vi "Begin.vi"(8 "error in":errorcluster) -> (0 "error out":errorcluster)   [LabVIEW 2019]
doc: "Called before other user functions, this VI is expected to open initial I/O refnums, load in file data, and do all program initialization. Notice that the <B>error out</B> terminal is simply used for data flow. Wiring it to other structures or subVIs ensures that this VI runs first."
uses:
  <vilib>/Rock Robotics/WPI/DriverStation/WPI_DriverStationRobotMode2.ctl
  <vilib>/Rock Robotics/WPI/Joystick/WPI_JoystickDeviceEnum.ctl
  Robot Global Data.vi
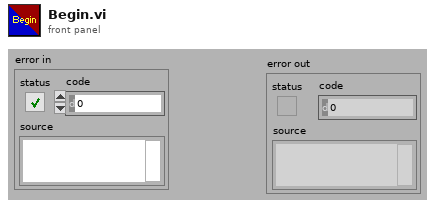
[diagram p1: front panel]
types:
  T1 = typedef "WPI_JoystickDeviceEnum.ctl" = enum16{"USB 0", "USB 1", "USB 2", "USB 3", "USB 4", "USB 5"}
  T2 = typedef "WPI_DriverStationRobotMode2.ctl" = enum16{"Autonomous Disabled", "Autonomous Enabled", "Teleop Disabled", "Teleop Enabled", "Disconnected", "Finish", "Test Disabled", "Test Enabled", "Emergency Stopped"}
  T3 = typedef "WPI_JoystickDevRef.ctl" = cluster{"Device":T1}
  T4 = typedef "WPI_MotorControlDeviceRef.ctl" = cluster{"DeviceStatus":errorcluster, "Type":T5, "PWM":cluster{"PWM Channel":T6, "DeadBand":T7}, "CAN":cluster{"Device Number":u8, "SetOutput VI Ref":variant, "GetOutput VI Ref":variant, "Enable VI Ref":variant, "Disable VI Ref":variant, "Data":variant}, "Invert":bool, "DIO PWM":cluster{"PWM \"Enable\" Channel":T6, "DIOChannel":T8, "PWM Rate":dbl}}
  T5 = typedef "WPI_MotorControlType.ctl" = enum16{"PWM", "CAN", "DIO PWM"}
  T6 = typedef "FPGA_DIOPWMChannel.ctl" = enum8{"PWM 0", "PWM 1", "PWM 2", "PWM 3", "PWM 4", "PWM 5", "PWM 6", "PWM 7", "PWM 8", "PWM 9", "PWM MXP 0", "PWM MXP 1", "PWM MXP 2", "PWM MXP 3", "PWM MXP 4", "PWM MXP 5", "PWM MXP 6", "PWM MXP 7", "PWM MXP 8", "PWM MXP 9", "Invalid"}
  T7 = typedef "WPI_PWMDeadband.ctl" = cluster{"Name":string, "maxPositivePwm":i32, "minPositivePwm":i32, "centerPwm":i32, "maxNegativePwm":i32, "minNegativePwm":i32, "angularRange":u16}
  T8 = typedef "FPGA_DIOChannel.ctl" = enum8{"DIO 0", "DIO 1", "DIO 2", "DIO 3", "DIO 4", "DIO 5", "DIO 6", "DIO 7", "DIO 8", "DIO 9", "DIO MXP 0", "DIO MXP 1", "DIO MXP 2", "DIO MXP 3", "DIO MXP 4", "DIO MXP 5", "DIO MXP 6", "DIO MXP 7", "DIO MXP 8", "DIO MXP 9", "DIO MXP 10", "DIO MXP 11", "DIO MXP 12", "DIO MXP 13", "DIO MXP 14", "DIO MXP 15", "SPI Port CS1", "SPI Port CS2", "SPI Port CS3", "SPI Port MISO", "SPI Port MOSI", "Invalid"}
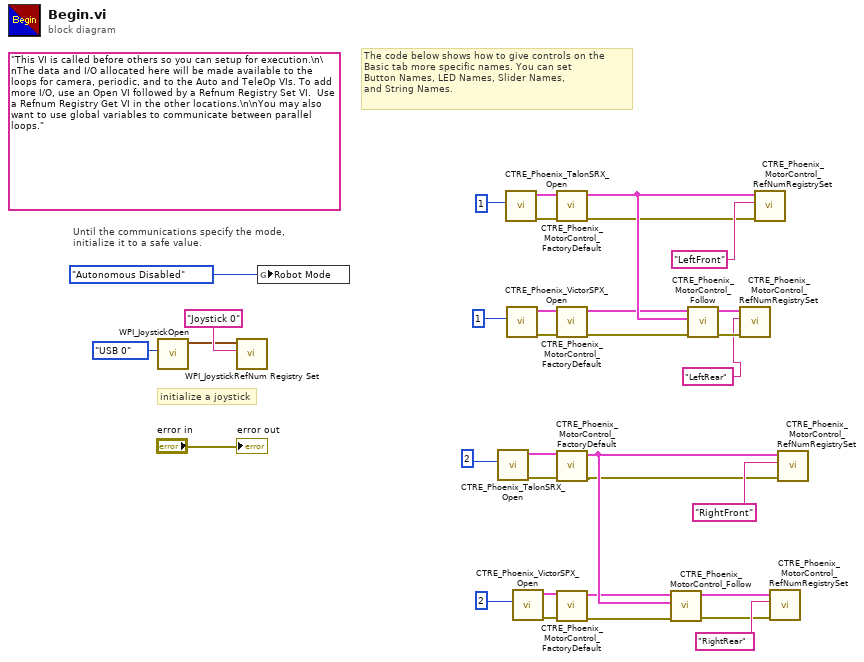
[diagram p0: block diagram]
diagram:
  (unwired) "This VI is called before others so you can setup for execution.\n\nThe data and I/O allocated here will be made available to the loops for camera, periodic, and to the Auto and TeleOp VIs. To add more I/O, use an Open VI followed by a Refnum Registry Set VI.  Use a Refnum Registry Get VI in the other locations.\n\nYou may also want to use global variables to communicate between parallel loops."
  # "The code below shows how to give controls on the\nBasic tab more specific names. You can set\nButton Names, LED Names, Slider Names,\nand String Names."
  # "initialize a joystick"
  # "Until the communications specify the mode,\ninitialize it to a safe value."
  n1 = call <vilib>:"WPI_JoystickOpen.vi"("JoystickDevice"=WPI_JoystickDeviceEnum."USB 0") -> ("JoystickDevRef"=w32:T3)  [unwired: 10 in]
  n2 = call <vilib>:"WPI_JoystickRefNum Registry Set.vi"("refnum name"="Joystick 0", "JoystickDevRef"=w32) -> ()  [unwired: 8 in, 2 out]
  n3 = global write "Robot Global Data.vi" "Robot Mode"(WPI_DriverStationRobotMode2."Autonomous Disabled" ("Robot Mode")) -> ()
  n4 = call <vilib>:"CTRE_Phoenix_TalonSRX_Open.vi"("Device Number"=u8 2) -> ("error out"=w5:errorcluster, "CAN Talon SRX Ref"=w15:T4)  [unwired: 9 in]
  n5 = call <vilib>:"CTRE_Phoenix_TalonSRX_Open.vi"("Device Number"=u8 1) -> ("error out"=w7:errorcluster, "CAN Talon SRX Ref"=w17:T4)  [unwired: 9 in]
  n6 = call <vilib>:"CTRE_Phoenix_VictorSPX_Open.vi"("Device Number"=u8 1) -> ("error out"=w9:errorcluster, "CAN Talon SRX Ref"=w11:T4)  [unwired: 9 in]
  n7 = call <vilib>:"CTRE_Phoenix_VictorSPX_Open.vi"("Device Number"=u8 2) -> ("error out"=w3:errorcluster, "CAN Talon SRX Ref"=w13:T4)  [unwired: 9 in]
  n8 = call <vilib>:"CTRE_Phoenix_MotorControl_FactoryDefault.vi"("error in"=w7, "PhoenixMotorControlDevRef"=w17) -> ("error out"=w6:errorcluster, "PhoenixMotorControlDevRef"=w16:T4)  [unwired: 8 in]
  n9 = call <vilib>:"CTRE_Phoenix_MotorControl_FactoryDefault.vi"("error in"=w9, "PhoenixMotorControlDevRef"=w11) -> ("error out"=w8:errorcluster, "PhoenixMotorControlDevRef"=w10:T4)  [unwired: 8 in]
  n10 = call <vilib>:"CTRE_Phoenix_MotorControl_FactoryDefault.vi"("error in"=w5, "PhoenixMotorControlDevRef"=w15) -> ("error out"=w4:errorcluster, "PhoenixMotorControlDevRef"=w14:T4)  [unwired: 8 in]
  n11 = call <vilib>:"CTRE_Phoenix_MotorControl_FactoryDefault.vi"("error in"=w3, "PhoenixMotorControlDevRef"=w13) -> ("error out"=w2:errorcluster, "PhoenixMotorControlDevRef"=w12:T4)  [unwired: 8 in]
  n12 = call <vilib>:"CTRE_Phoenix_MotorControl_Follow.vi"("error in (no error)"=w2, "Master Controller to Follow"=w14, "PhoenixMotorControlDevRef"=w12) -> ("error out"=w19:errorcluster, "PhoenixMotorControlDevRef"=w18:T4)  [unwired: 7 in]
  n13 = call <vilib>:"CTRE_Phoenix_MotorControl_Follow.vi"("error in (no error)"=w8, "Master Controller to Follow"=w16, "PhoenixMotorControlDevRef"=w10) -> ("error out"=w27:errorcluster, "PhoenixMotorControlDevRef"=w26:T4)  [unwired: 7 in]
  n14 = call <vilib>:"CTRE_Phoenix_MotorControl_RefNumRegistrySet.vi"("error in (no error)"=w27, "refnum name"="LeftRear", "PhoenixMotorControlDevRef"=w26) -> ()  [unwired: 7 in, 2 out]
  n15 = call <vilib>:"CTRE_Phoenix_MotorControl_RefNumRegistrySet.vi"("error in (no error)"=w6, "refnum name"="LeftFront", "PhoenixMotorControlDevRef"=w16) -> ()  [unwired: 7 in, 2 out]
  n16 = call <vilib>:"CTRE_Phoenix_MotorControl_RefNumRegistrySet.vi"("error in (no error)"=w19, "refnum name"="RightRear", "PhoenixMotorControlDevRef"=w18) -> ()  [unwired: 7 in, 2 out]
  n17 = call <vilib>:"CTRE_Phoenix_MotorControl_RefNumRegistrySet.vi"("error in (no error)"=w4, "refnum name"="RightFront", "PhoenixMotorControlDevRef"=w14) -> ()  [unwired: 7 in, 2 out]
  "error out" <- "error in"
